vi "215.Errors (SubVI).vi"(8 "error in (no error)":errorcluster, 11 "VISA resource name":refnum<visa-resource-name>="COM7") -> (0 "error out":errorcluster, 1 "String":string, 2 "Connected":bool, 3 "VISA Out":refnum<visa-resource-name>)   [LabVIEW 2020]
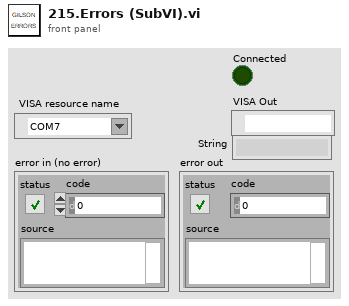
[diagram p1: front panel]
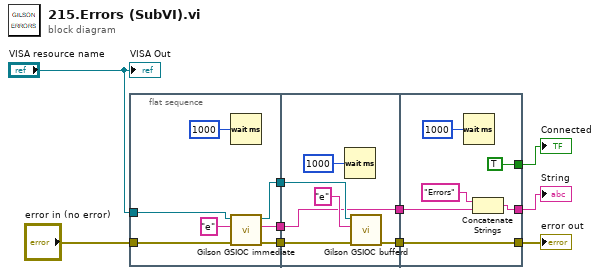
[diagram p0: block diagram]
diagram:
  n1 = flat-sequence {
    tunnel: "VISA resource name" -> [w15]
    tunnel: "error in (no error)" -> [w17]
    tunnel: [w14] -> w10
    tunnel: [w13] -> w9
    tunnel: [w11] -> w7
    tunnel: w10 -> [w23]
    tunnel: w9 -> [w21]
    tunnel: w7 -> [w19]
    tunnel: [w19] -> w2
    tunnel: [w18] -> w1
    tunnel: [TRUE ("Connected")] -> w8
    tunnel: w2 -> [w28]
    tunnel: [w24] -> w6
    tunnel: [w26] -> w5
    tunnel: w1 -> [w24]
    frame #0 {
      n2 = Wait (ms)(milliseconds to wait=u32 1000) -> ()  [unwired: 1 out]
      n3 = call <instrlib>:"Gilson GSIOC immediate.vi"("error in (no error)"=w17, "Immediate command"="e", "VISA resource name"=w15) -> ("error out"=w13:errorcluster, "Receive string"=w11:string, "VISA resource name"=w14:refnum<visa-resource-name>)  [unwired: 6 in]
    }
    frame #1 {
      n4 = Wait (ms)(milliseconds to wait=u32 1000) -> ()  [unwired: 1 out]
      n5 = call <instrlib>:"Gilson GSIOC bufferd.vi"("error in (no error)"=w21, "Bufferd command"="e", "VISA resource name"=w23) -> ("error out"=w18:errorcluster)  [unwired: 6 in, 2 out]
    }
    frame #2 {
      n6 = Wait (ms)(milliseconds to wait=u32 1000) -> ()  [unwired: 1 out]
      n7 = Concatenate Strings("Errors" ("string"), w28) -> (w26:string)
    }
  }
  "VISA Out" <- "VISA resource name"
  "error out" <- w6
  "Connected" <- w8
  "String" <- w5
